vi "Zero Yields.vi"(8 "error in (no error)":errorcluster, 11 "Master in":refnum<class "Master.lvclass">) -> (0 "error out":errorcluster, 3 "Master out":refnum<class "Master.lvclass">)   [LabVIEW 2014, in "Master.lvclass"]
uses:
  Master/Master.lvclass
  Master/Master.lvclass/Master.ctl
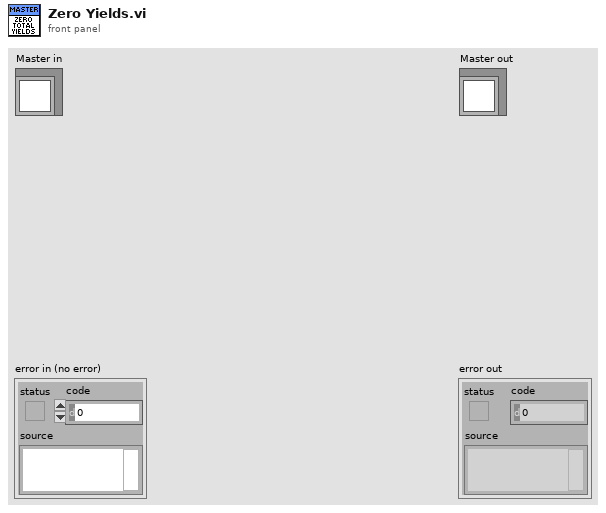
[diagram p1: front panel]
types:
  T1 = cluster{"Production Record":cluster{"User":string, "Date":string, "Yields":dbl, "hour":i32, "minute":i32}[], "Total Yields":dbl}
  T2 = cluster{"User":string, "Date":string, "Yields":dbl, "hour":i32, "minute":i32}[]
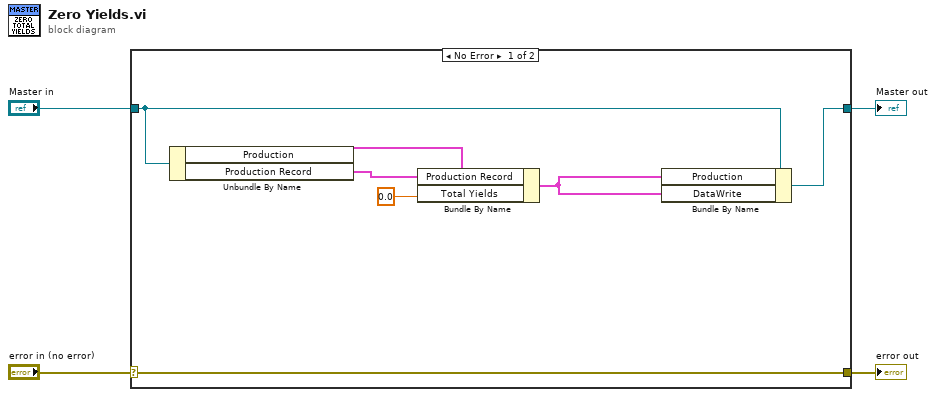
[diagram p0: block diagram]
diagram:
  n1 = case shown="No Error" "error in (no error)" {
    selector: "error in (no error)" -> [w11 w13]
    tunnel: [w11 w13] -> w3
    tunnel: [w10 w12] -> w1
    tunnel: "Master in" -> [w9 w12]
    frame No Error {
      n2 = Unbundle By Name(w9) -> ("Production"=w8:T1, "Production Record"=w7:T2)
      n3 = Bundle By Name(cluster=w8, "Production Record"=w7, "Total Yields"=0.0) -> (w5:T1)
      n4 = Bundle By Name(cluster=w9, "Production"=w5, "DataWrite"=w5) -> (w10:refnum<class "Master.lvclass">)
    }
    frame Error {
    }
  }
  "error out" <- w3
  "Master out" <- w1
